vi "Read Wiring Configuration.vi"(8 "error in (no error)":errorcluster, 11 "Control Experiment":refnum<class "Control Experiment.lvclass">) -> (0 "error out":errorcluster, 2 "Wiring Configuration":T1, 3 "Control Experiment out":refnum<class "Control Experiment.lvclass">)   [LabVIEW 2016, in "Control Experiment.lvclass"]
uses:
  Control Experiment.lvclass
  Typedefs/Wiring Description--cluster.ctl
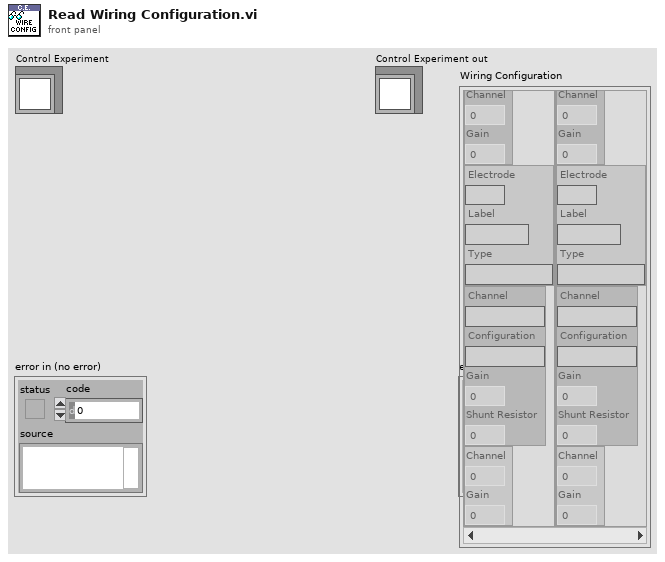
[diagram p1: front panel]
types:
  T1 = typedef "Control Experiment.lvclass/Wiring Description--cluster.ctl" = cluster{"AI":cluster{"Channel":u32, "Gain":dbl}, "Device":cluster{"Electrode":string, "Label":string, "Type":string}, "KH":cluster{"Channel":string, "Configuration":string, "Gain":u32, "Shunt Resistor":u32}, "AO":cluster{"Channel":u32, "Gain":dbl}}[]
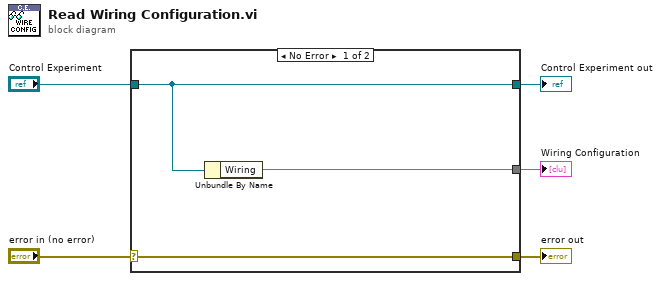
[diagram p0: block diagram]
diagram:
  n1 = case shown="No Error" "error in (no error)" {
    selector: "error in (no error)" -> [w8 w9]
    tunnel: [w8 w9] -> w4
    tunnel: [w7 w10] -> w2
    tunnel: "Control Experiment" -> [w7 w10]
    tunnel: [w6 _] -> w1
    frame No Error {
      n2 = Unbundle By Name(w7) -> ("Wiring"=w6)
    }
    frame Error {
    }
  }
  "error out" <- w4
  "Control Experiment out" <- w2
  "Wiring Configuration" <- w1
